vi "Viewer.vi"(8 "error in (no error)":errorcluster) -> (0 "error out":errorcluster)   [LabVIEW 2014]
uses:
  TableLogger_Actor/TableLogger_Actor/TableLogger_Actor.lvclass
  <vilib>/ActorFramework/Stop Msg/Stop Msg.lvclass
  TableLogger_Actor/Messages/InsertData_Msg/InsertData Msg.lvclass
  TableLogger_Actor/TableLoggerTypes.ctl
  TableLogger_Actor/TableLogger_Actor.lvlib
  TableLogger_Actor/TableLoggerBackupConfig.ctl
  TableLogger_Actor/TableLoggerConfig.ctl
  TableLogger_CSV_Actor/TableLogger_CSV_Actor/TableLogger_CSV_Actor.lvclass
  TableLogger_SQLite_Actor/TableLogger_SQLite_Actor/TableLogger_SQLite_Actor.lvclass
panel:
  # "Look at the block diagram for details about this VI"
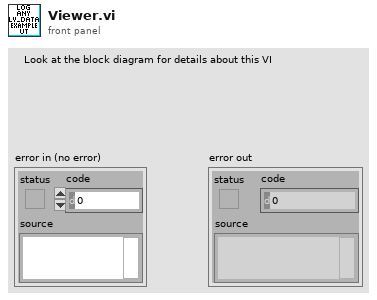
[diagram p1: front panel]
types:
  T1 = enum16{"Poll", "Initialize", "Insert Data", "Update ", "Select", "Delete", "Stop", "Abort"}
  T2 = typedef "TableLogger_Actor.lvlib/TableLoggerConfig.ctl" = cluster{"TableLogger":T3, "DB File Path":path, "DB Backup Config":T4}
  T3 = typedef "TableLogger_Actor.lvlib/TableLoggerTypes.ctl" = enum16{"CSV Logger", "SQLite Logger"}
  T4 = typedef "TableLogger_Actor.lvlib/TableLoggerBackupConfig.ctl" = cluster{"Directory":path, "UTC Time Format":bool, "On Launch":bool, "Interval (Hours)":dbl, "Size Multiples (Bytes)":i32}
  T5 = cluster{"Numeric Data":i32, "Float Data":dbl, "String Data":string, "Enum Data":enum16{"Enum Item 1", "Enum Item 2"}}
  T6 = cluster{"Numeric Data":i32, "Float Data":dbl, "String Data":string, "Enum Data":enum16{"Enum Item 1", "Enum Item 2"}, "Array Data 2":i32[], "Cluster 2":cluster{"String":string, "Array Data 2":i32[]}, "Cluster 3":cluster{"Cluster78":cluster{"Array Data 2":i32[]}}, "Enum Data 2":enum16{"Enum Item 1", "Enum Item 2"}, "String Data 2":string, "Float Data 2":dbl, "Array Data":i32[], "Array A":cluster{"String A":string, "Array B":cluster{"String B":string, "Array B 2":cluster{"String B":string}[]}[], "Array B 2":cluster{"String B":string}[]}[]}[]
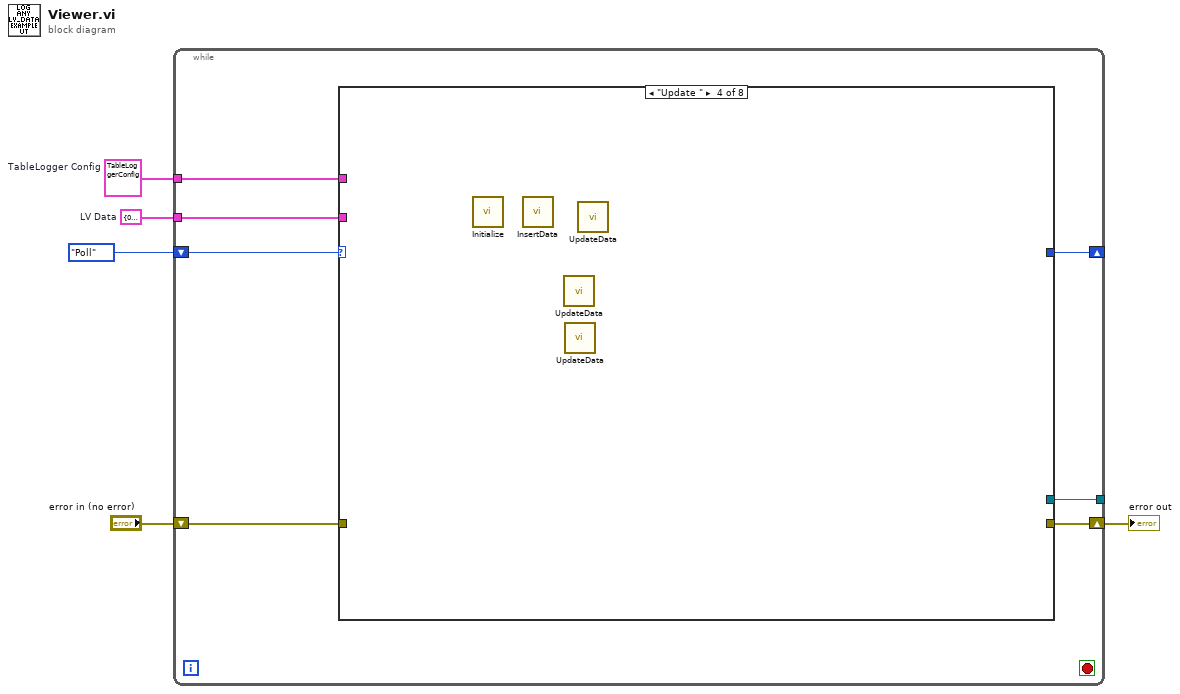
[diagram p0: block diagram]
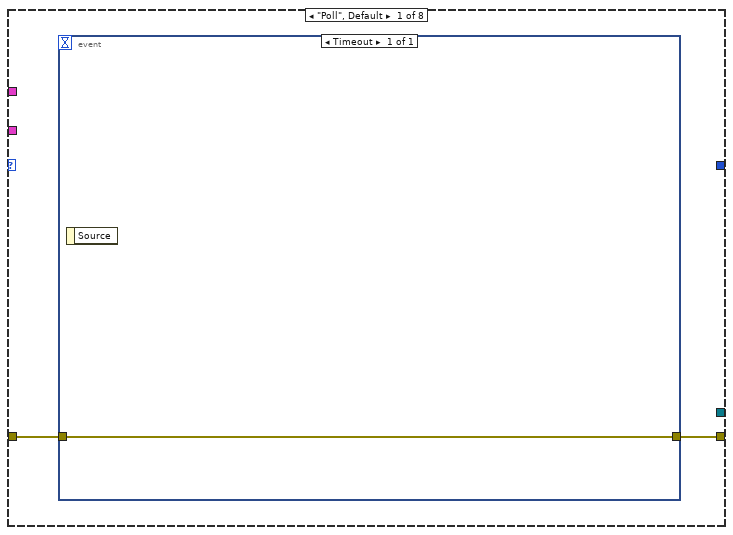
[diagram p2: hidden frame]
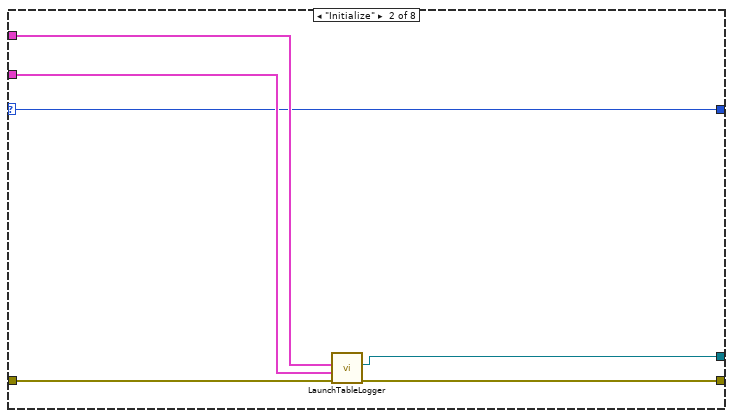
[diagram p3: hidden frame]
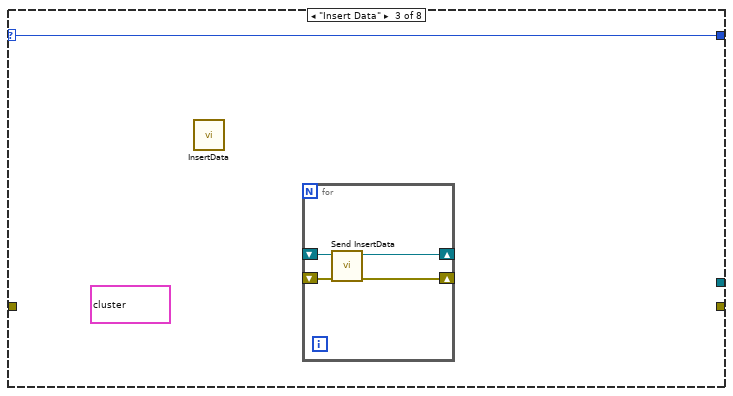
[diagram p4: hidden frame]
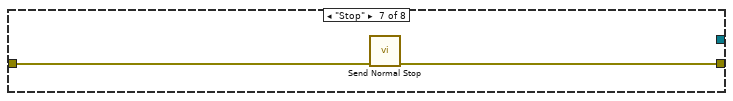
[diagram p7: hidden frame]
diagram:
  w4 = T2 {"TableLogger"=enum."SQLite Logger", "DB File Path"=path "C:/LogAnyLVdata/Test.db", "DB Backup Config"={"Directory"=path "C:/LogAnyLVdata/dBbackup", "UTC Time Format"=FALSE, "On Launch"=TRUE, "Interval (Hours)"=-1.0, "Size Multiples (Bytes)"=10000}}  # TableLogger Config
  w3 = T5 {"Numeric Data"=0, "Float Data"=0.0, "String Data"="", "Enum Data"=enum."Enum Item 2"}  # LV Data
  n1 = while {
    tunnel: [w12] -> _
    tunnel: w4 -> [w9]
    tunnel: w3 -> [w8]
    shift-right: [w11] -> w2
    shift-left: "error in (no error)" -> [w10]
    shift-right: [w6] -> _
    shift-left: T1."Poll" -> [w7]
    stop <- _ stop-if-true
    n2 = case shown="\"Update \"" w7 {
      selector: w7 -> [_ w16 w22 _ _ _ _ _]
      tunnel: [_ w21 _ _ _ _ _ _] -> w12
      tunnel: [w14 w20 _ _ _ _ w27 _] -> w11
      tunnel: w10 -> [w13 w19 _ _ _ _ w28 _]
      tunnel: w9 -> [_ w18 _ _ _ _ _ _]
      tunnel: w8 -> [_ w17 _ _ _ _ _ _]
      tunnel: [_ w16 w22 _ _ _ _ _] -> w6
      frame "Poll", Default {
        n3 = event shown="[0] Timeout" {
          selector: _ -> [_]
          dyn-events: _ -> [_]
          timeout: _ -> [_]
          tunnel: [w15] -> w14
          tunnel: w13 -> [w15]
          event Timeout {
            n4 = event-data() -> ()  [unwired: 1 in, 1 out]
          }
        }
      }
      frame "Initialize" {
        n5 = call "LaunchTableLogger.vi"("error in (no error)"=w19, "Data Cluster (for Headers)"=w17, "TableLogger Config"=w18) -> ("error out"=w20:errorcluster, "TableLogger Actor's Enqueuer"=w21:refnum<class "Message Enqueuer.lvclass">)  [unwired: 5 in, 2 out]
      }
      frame "Insert Data" {
        (unwired) T6 [{"Numeric Data"=0, "Float Data"=0.0, "String Data"="", "Enum Data"=enum."Enum Item 1", "Array Data 2"=[0, 0, 0], "Cluster 2"={"String"="", "Array Data 2"=[0, 0, 0]}, "Cluster 3"={"Cluster78"={"Array Data 2"=[0, 0, 0]}}, "Enum Data 2"=enum."Enum Item 1", "String Data 2"="", "Float Data 2"=0.0, "Array Data"=[0, 0, 0, 4], "Array A"=[{"String A"="hello", "Array B"=[{"String B"="uq", "Array B 2"=[{"String B"="u"}, {"String B"="c"}, {"String B"="hello"}]}, {"String B"="c", "Array B 2"=[{"String B"="u"}, {"String B"="c"}, {"String B"="hello"}]}, {"String B"="hello", "Array B 2"=[{"String B"="u"}, {"String B"="c"}, {"String B"="hello"}]}], "Array B 2"=[{"String B"="u"}, {"String B"="c"}, {"String B"="hello"}]}, {"String A"="hello", "Array B"=[{"String B"="uP", "Array B 2"=[{"String B"="u"}, {"String B"="c"}, {"String B"="hello"}]}, {"String B"="c", "Array B 2"=[{"String B"="u"}, {"String B"="c"}, {"String B"="hello"}]}, {"String B"="hello", "Array B 2"=[{"String B"="u"}, {"String B"="c"}, {"String B"="hello"}]}], "Array B 2"=[{"String B"="u"}, {"String B"="c"}, {"String B"="hello"}]}]}, {"Numeric Data"=401, "Float Data"=0.0, "String Data"="q", "Enum Data"=enum."Enum Item 1", "Array Data 2"=[0, 0, 0], "Cluster 2"={"String"="", "Array Data 2"=[0, 0, 0]}, "Cluster 3"={"Cluster78"={"Array Data 2"=[0, 0, 0]}}, "Enum Data 2"=enum."Enum Item 1", "String Data 2"="", "Float Data 2"=0.0, "Array Data"=[0, 0, 0, 4], "Array A"=[{"String A"="hello", "Array B"=[{"String B"="uq", "Array B 2"=[{"String B"="u"}, {"String B"="c"}, {"String B"="hello"}]}, {"String B"="c", "Array B 2"=[{"String B"="u"}, {"String B"="c"}, {"String B"="hello"}]}, {"String B"="hello", "Array B 2"=[{"String B"="u"}, {"String B"="c"}, {"String B"="hello"}]}], "Array B 2"=[{"String B"="u"}, {"String B"="c"}, {"String B"="hello"}]}, {"String A"="hello", "Array B"=[{"String B"="uP", "Array B 2"=[{"String B"="u"}, {"String B"="c"}, {"String B"="hello"}]}, {"String B"="c", "Array B 2"=[{"String B"="u"}, {"String B"="c"}, {"String B"="hello"}]}, {"String B"="hello", "Array B 2"=[{"String B"="u"}, {"String B"="c"}, {"String B"="hello"}]}], "Array B 2"=[{"String B"="u"}, {"String B"="c"}, {"String B"="hello"}]}]}, {"Numeric Data"=0, "Float Data"=0.0, "String Data"="", "Enum Data"=enum."Enum Item 1", "Array Data 2"=[0, 0, 0], "Cluster 2"={"String"="", "Array Data 2"=[0, 0, 0]}, "Cluster 3"={"Cluster78"={"Array Data 2"=[0, 0, 0]}}, "Enum Data 2"=enum."Enum Item 1", "String Data 2"="", "Float Data 2"=0.0, "Array Data"=[0, 0, 0, 4], "Array A"=[{"String A"="hello", "Array B"=[{"String B"="uq", "Array B 2"=[{"String B"="u"}, {"String B"="c"}, {"String B"="hello"}]}, {"String B"="c", "Array B 2"=[{"String B"="u"}, {"String B"="c"}, {"String B"="hello"}]}, {"String B"="hello", "Array B 2"=[{"String B"="u"}, {"String B"="c"}, {"String B"="hello"}]}], "Array B 2"=[{"String B"="u"}, {"String B"="c"}, {"String B"="hello"}]}, {"String A"="hello", "Array B"=[{"String B"="uP", "Array B 2"=[{"String B"="u"}, {"String B"="c"}, {"String B"="hello"}]}, {"String B"="c", "Array B 2"=[{"String B"="u"}, {"String B"="c"}, {"String B"="hello"}]}, {"String B"="hello", "Array B 2"=[{"String B"="u"}, {"String B"="c"}, {"String B"="hello"}]}], "Array B 2"=[{"String B"="u"}, {"String B"="c"}, {"String B"="hello"}]}]}, {"Numeric Data"=0, "Float Data"=0.0, "String Data"="", "Enum Data"=enum."Enum Item 1", "Array Data 2"=[0, 0, 0], "Cluster 2"={"String"="", "Array Data 2"=[0, 0, 0]}, "Cluster 3"={"Cluster78"={"Array Data 2"=[0, 0, 0]}}, "Enum Data 2"=enum."Enum Item 1", "String Data 2"="", "Float Data 2"=0.0, "Array Data"=[0, 0, 0, 4], "Array A"=[{"String A"="hello", "Array B"=[{"String B"="uq", "Array B 2"=[{"String B"="u"}, {"String B"="c"}, {"String B"="hello"}]}, {"String B"="c", "Array B 2"=[{"String B"="u"}, {"String B"="c"}, {"String B"="hello"}]}, {"String B"="hello", "Array B 2"=[{"String B"="u"}, {"String B"="c"}, {"String B"="hello"}]}], "Array B 2"=[{"String B"="u"}, {"String B"="c"}, {"String B"="hello"}]}, {"String A"="hello", "Array B"=[{"String B"="uP", "Array B 2"=[{"String B"="u"}, {"String B"="c"}, {"String B"="hello"}]}, {"String B"="c", "Array B 2"=[{"String B"="u"}, {"String B"="c"}, {"String B"="hello"}]}, {"String B"="hello", "Array B 2"=[{"String B"="u"}, {"String B"="c"}, {"String B"="hello"}]}], "Array B 2"=[{"String B"="u"}, {"String B"="c"}, {"String B"="hello"}]}]}, {"Numeric Data"=0, "Float Data"=0.0, "String Data"="", "Enum Data"=enum."Enum Item 1", "Array Data 2"=[0, 0, 0], "Cluster 2"={"String"="", "Array Data 2"=[0, 0, 0]}, "Cluster 3"={"Cluster78"={"Array Data 2"=[0, 0, 0]}}, "Enum Data 2"=enum."Enum Item 1", "String Data 2"="", "Float Data 2"=0.0, "Array Data"=[0, 0, 0, 4], "Array A"=[{"String A"="hello", "Array B"=[{"String B"="uq", "Array B 2"=[{"String B"="u"}, {"String B"="c"}, {"String B"="hello"}]}, {"String B"="c", "Array B 2"=[{"String B"="u"}, {"String B"="c"}, {"String B"="hello"}]}, {"String B"="hello", "Array B 2"=[{"String B"="u"}, {"String B"="c"}, {"String B"="hello"}]}], "Array B 2"=[{"String B"="u"}, {"String B"="c"}, {"String B"="hello"}]}, {"String A"="hello", "Array B"=[{"String B"="uP", "Array B 2"=[{"String B"="u"}, {"String B"="c"}, {"String B"="hello"}]}, {"String B"="c", "Array B 2"=[{"String B"="u"}, {"String B"="c"}, {"String B"="hello"}]}, {"String B"="hello", "Array B 2"=[{"String B"="u"}, {"String B"="c"}, {"String B"="hello"}]}], "Array B 2"=[{"String B"="u"}, {"String B"="c"}, {"String B"="hello"}]}]}, {"Numeric Data"=0, "Float Data"=0.0, "String Data"="", "Enum Data"=enum."Enum Item 1", "Array Data 2"=[0, 0, 0], "Cluster 2"={"String"="", "Array Data 2"=[0, 0, 0]}, "Cluster 3"={"Cluster78"={"Array Data 2"=[0, 0, 0]}}, "Enum Data 2"=enum."Enum Item 1", "String Data 2"="", "Float Data 2"=0.0, "Array Data"=[0, 0, 0, 4], "Array A"=[{"String A"="hello", "Array B"=[{"String B"="uq", "Array B 2"=[{"String B"="u"}, {"String B"="c"}, {"String B"="hello"}]}, {"String B"="c", "Array B 2"=[{"String B"="u"}, {"String B"="c"}, {"String B"="hello"}]}, {"String B"="hello", "Array B 2"=[{"String B"="u"}, {"String B"="c"}, {"String B"="hello"}]}], "Array B 2"=[{"String B"="u"}, {"String B"="c"}, {"String B"="hello"}]}, {"String A"="hello", "Array B"=[{"String B"="uP", "Array B 2"=[{"String B"="u"}, {"String B"="c"}, {"String B"="hello"}]}, {"String B"="c", "Array B 2"=[{"String B"="u"}, {"String B"="c"}, {"String B"="hello"}]}, {"String B"="hello", "Array B 2"=[{"String B"="u"}, {"String B"="c"}, {"String B"="hello"}]}], "Array B 2"=[{"String B"="u"}, {"String B"="c"}, {"String B"="hello"}]}]}, {"Numeric Data"=0, "Float Data"=0.0, "String Data"="", "Enum Data"=enum."Enum Item 1", "Array Data 2"=[0, 0, 0], "Cluster 2"={"String"="", "Array Data 2"=[0, 0, 0]}, "Cluster 3"={"Cluster78"={"Array Data 2"=[0, 0, 0]}}, "Enum Data 2"=enum."Enum Item 1", "String Data 2"="", "Float Data 2"=0.0, "Array Data"=[0, 0, 0, 4], "Array A"=[{"String A"="hello", "Array B"=[{"String B"="uq", "Array B 2"=[{"String B"="u"}, {"String B"="c"}, {"String B"="hello"}]}, {"String B"="c", "Array B 2"=[{"String B"="u"}, {"String B"="c"}, {"String B"="hello"}]}, {"String B"="hello", "Array B 2"=[{"String B"="u"}, {"String B"="c"}, {"String B"="hello"}]}], "Array B 2"=[{"String B"="u"}, {"String B"="c"}, {"String B"="hello"}]}, {"String A"="hello", "Array B"=[{"String B"="uP", "Array B 2"=[{"String B"="u"}, {"String B"="c"}, {"String B"="hello"}]}, {"String B"="c", "Array B 2"=[{"String B"="u"}, {"String B"="c"}, {"String B"="hello"}]}, {"String B"="hello", "Array B 2"=[{"String B"="u"}, {"String B"="c"}, {"String B"="hello"}]}], "Array B 2"=[{"String B"="u"}, {"String B"="c"}, {"String B"="hello"}]}]}, {"Numeric Data"=0, "Float Data"=0.0, "String Data"="", "Enum Data"=enum."Enum Item 1", "Array Data 2"=[0, 0, 0], "Cluster 2"={"String"="", "Array Data 2"=[0, 0, 0]}, "Cluster 3"={"Cluster78"={"Array Data 2"=[0, 0, 0]}}, "Enum Data 2"=enum."Enum Item 1", "String Data 2"="", "Float Data 2"=0.0, "Array Data"=[0, 0, 0, 4], "Array A"=[{"String A"="hello", "Array B"=[{"String B"="uq", "Array B 2"=[{"String B"="u"}, {"String B"="c"}, {"String B"="hello"}]}, {"String B"="c", "Array B 2"=[{"String B"="u"}, {"String B"="c"}, {"String B"="hello"}]}, {"String B"="hello", "Array B 2"=[{"String B"="u"}, {"String B"="c"}, {"String B"="hello"}]}], "Array B 2"=[{"String B"="u"}, {"String B"="c"}, {"String B"="hello"}]}, {"String A"="hello", "Array B"=[{"String B"="uP", "Array B 2"=[{"String B"="u"}, {"String B"="c"}, {"String B"="hello"}]}, {"String B"="c", "Array B 2"=[{"String B"="u"}, {"String B"="c"}, {"String B"="hello"}]}, {"String B"="hello", "Array B 2"=[{"String B"="u"}, {"String B"="c"}, {"String B"="hello"}]}], "Array B 2"=[{"String B"="u"}, {"String B"="c"}, {"String B"="hello"}]}]}, {"Numeric Data"=0, "Float Data"=0.0, "String Data"="", "Enum Data"=enum."Enum Item 1", "Array Data 2"=[0, 0, 0], "Cluster 2"={"String"="", "Array Data 2"=[0, 0, 0]}, "Cluster 3"={"Cluster78"={"Array Data 2"=[0, 0, 0]}}, "Enum Data 2"=enum."Enum Item 1", "String Data 2"="", "Float Data 2"=0.0, "Array Data"=[0, 0, 0, 4], "Array A"=[{"String A"="hello", "Array B"=[{"String B"="uq", "Array B 2"=[{"String B"="u"}, {"String B"="c"}, {"String B"="hello"}]}, {"String B"="c", "Array B 2"=[{"String B"="u"}, {"String B"="c"}, {"String B"="hello"}]}, {"String B"="hello", "Array B 2"=[{"String B"="u"}, {"String B"="c"}, {"String B"="hello"}]}], "Array B 2"=[{"String B"="u"}, {"String B"="c"}, {"String B"="hello"}]}, {"String A"="hello", "Array B"=[{"String B"="uP", "Array B 2"=[{"String B"="u"}, {"String B"="c"}, {"String B"="hello"}]}, {"String B"="c", "Array B 2"=[{"String B"="u"}, {"String B"="c"}, {"String B"="hello"}]}, {"String B"="hello", "Array B 2"=[{"String B"="u"}, {"String B"="c"}, {"String B"="hello"}]}], "Array B 2"=[{"String B"="u"}, {"String B"="c"}, {"String B"="hello"}]}]}, {"Numeric Data"=0, "Float Data"=0.0, "String Data"="", "Enum Data"=enum."Enum Item 1", "Array Data 2"=[0, 0, 0], "Cluster 2"={"String"="", "Array Data 2"=[0, 0, 0]}, "Cluster 3"={"Cluster78"={"Array Data 2"=[0, 0, 0]}}, "Enum Data 2"=enum."Enum Item 1", "String Data 2"="", "Float Data 2"=0.0, "Array Data"=[0, 0, 0, 4], "Array A"=[{"String A"="hello", "Array B"=[{"String B"="uq", "Array B 2"=[{"String B"="u"}, {"String B"="c"}, {"String B"="hello"}]}, {"String B"="c", "Array B 2"=[{"String B"="u"}, {"String B"="c"}, {"String B"="hello"}]}, {"String B"="hello", "Array B 2"=[{"String B"="u"}, {"String B"="c"}, {"String B"="hello"}]}], "Array B 2"=[{"String B"="u"}, {"String B"="c"}, {"String B"="hello"}]}, {"String A"="hello", "Array B"=[{"String B"="uP", "Array B 2"=[{"String B"="u"}, {"String B"="c"}, {"String B"="hello"}]}, {"String B"="c", "Array B 2"=[{"String B"="u"}, {"String B"="c"}, {"String B"="hello"}]}, {"String B"="hello", "Array B 2"=[{"String B"="u"}, {"String B"="c"}, {"String B"="hello"}]}], "Array B 2"=[{"String B"="u"}, {"String B"="c"}, {"String B"="hello"}]}]}, {"Numeric Data"=0, "Float Data"=0.0, "String Data"="", "Enum Data"=enum."Enum Item 1", "Array Data 2"=[0, 0, 0], "Cluster 2"={"String"="", "Array Data 2"=[0, 0, 0]}, "Cluster 3"={"Cluster78"={"Array Data 2"=[0, 0, 0]}}, "Enum Data 2"=enum."Enum Item 1", "String Data 2"="", "Float Data 2"=0.0, "Array Data"=[0, 0, 0, 4], "Array A"=[{"String A"="hello", "Array B"=[{"String B"="uq", "Array B 2"=[{"String B"="u"}, {"String B"="c"}, {"String B"="hello"}]}, {"String B"="c", "Array B 2"=[{"String B"="u"}, {"String B"="c"}, {"String B"="hello"}]}, {"String B"="hello", "Array B 2"=[{"String B"="u"}, {"String B"="c"}, {"String B"="hello"}]}], "Array B 2"=[{"String B"="u"}, {"String B"="c"}, {"String B"="hello"}]}, {"String A"="hello", "Array B"=[{"String B"="uP", "Array B 2"=[{"String B"="u"}, {"String B"="c"}, {"String B"="hello"}]}, {"String B"="c", "Array B 2"=[{"String B"="u"}, {"String B"="c"}, {"String B"="hello"}]}, {"String B"="hello", "Array B 2"=[{"String B"="u"}, {"String B"="c"}, {"String B"="hello"}]}], "Array B 2"=[{"String B"="u"}, {"String B"="c"}, {"String B"="hello"}]}]}, {"Numeric Data"=401, "Float Data"=0.0, "String Data"="", "Enum Data"=enum."Enum Item 1", "Array Data 2"=[0, 0, 0], "Cluster 2"={"String"="", "Array Data 2"=[0, 0, 0]}, "Cluster 3"={"Cluster78"={"Array Data 2"=[0, 0, 0]}}, "Enum Data 2"=enum."Enum Item 1", "String Data 2"="", "Float Data 2"=0.0, "Array Data"=[0, 0, 0, 4], "Array A"=[{"String A"="hello", "Array B"=[{"String B"="uq", "Array B 2"=[{"String B"="u"}, {"String B"="c"}, {"String B"="hello"}]}, {"String B"="c", "Array B 2"=[{"String B"="u"}, {"String B"="c"}, {"String B"="hello"}]}, {"String B"="hello", "Array B 2"=[{"String B"="u"}, {"String B"="c"}, {"String B"="hello"}]}], "Array B 2"=[{"String B"="u"}, {"String B"="c"}, {"String B"="hello"}]}, {"String A"="hello", "Array B"=[{"String B"="uP", "Array B 2"=[{"String B"="u"}, {"String B"="c"}, {"String B"="hello"}]}, {"String B"="c", "Array B 2"=[{"String B"="u"}, {"String B"="c"}, {"String B"="hello"}]}, {"String B"="hello", "Array B 2"=[{"String B"="u"}, {"String B"="c"}, {"String B"="hello"}]}], "Array B 2"=[{"String B"="u"}, {"String B"="c"}, {"String B"="hello"}]}]}]
        n6 = call-dynamic "InsertData.vi"() -> ()  [unwired: 10 in, 2 out]
        n7 = for {
          shift-right: [w23] -> _
          shift-left: _ -> [w26]
          shift-right: [w24] -> _
          shift-left: _ -> [w25]
          n8 = call "Send InsertData.vi"("error in (no error)"=w25, "Message Enqueuer"=w26) -> ("error out"=w24:errorcluster, "Message Enqueuer out"=w23:refnum<class "Message Enqueuer.lvclass">)  [unwired: 8 in]
        }
      }
      frame "Update " {
        n9 = call-dynamic "Initialize.vi"() -> ()  [unwired: 10 in, 2 out]
        n10 = call-dynamic "InsertData.vi"() -> ()  [unwired: 10 in, 2 out]
        n11 = call-dynamic "UpdateData.vi"() -> ()  [unwired: 9 in, 3 out]
        n12 = call-dynamic "UpdateData.vi"() -> ()  [unwired: 9 in, 3 out]
        n13 = call-dynamic "UpdateData.vi"() -> ()  [unwired: 9 in, 3 out]
      }
      frame "Select" {
      }
      frame "Delete" {
      }
      frame "Stop" {
        n14 = call <vilib>:"Send Normal Stop.vi"("error in (no error)"=w28) -> ("error out"=w27:errorcluster)  [unwired: 10 in]
      }
      frame "Abort" {
      }
    }
  }
  "error out" <- w2
